vi "Get Output DMA Refs.vi"(8 "error in (no error)":errorcluster, 9 "FPGA Ref":refnum<k20>, 10 "Item GUID":string, 11 "Section Ref in":T7 format="%.0x") -> (0 "error out":errorcluster, 1 "FPGA Ref":refnum<k20>, 2 "DMA":T1[](array[typedef]) {"DMA Settings"."dt" format="%#_p"; "DMA Settings"."Update Rate" items=["1 Hz"=1, "2 Hz"=2, "5 Hz"=5, "10 Hz"=10]; "Refs"."Pairs"."Refs" format="%.0x"}, 3 "Section Ref out":T7 format="%.0x")   [LabVIEW 2013, in "FPGA Addon Engine.lvlib"]
uses:
  FPGA Addon Engine.lvlib
  <vilib>/NI Veristand/Custom Device API/Custom Device Item Ref.ctl
  Types/DMA Output Settings.ctl
  Inline Async API/Controls/Write To VS Engine.ctl
  <vilib>/NI Veristand/Custom Device API/Data Reference.ctl
  Types/DMA Output Ref.ctl
  <vilib>/NI VeriStand/Custom Device Waveform API/Single Waveform Read (DBL)/Single Waveform Read (DBL).lvclass
  Shared/DMA Settings.ctl
  Shared/Delacing Scheme.ctl
  Shared/FG Action.ctl
  <vilib>/NI/LVFPGA Adv Session Resources/OpenByNameSubVI.vi
  <vilib>/rvi/interface/common/niFpgaWaitOnOcc.vi
  <vilib>/NI Veristand/Custom Device Tools/Custom Device Utility Library/NI VeriStand - Search for Item by GUID.vi
  Shared/Constants.vi
  <vilib>/NI Veristand/Custom Device API/Get Item Property (Variant).vi
  <vilib>/NI Veristand/Custom Device Tools/Custom Device Utility Library/NI VeriStand - Search for All Items by GUID.vi
  <vilib>/NI Veristand/Custom Device API/Get Item Property (String).vi
  <vilib>/NI Veristand/Custom Device Waveform API/Single Waveform Read (DBL)/NI VeriStand - Open Single Waveform Read Session (DBL).vi
  <vilib>/NI Veristand/Custom Device API/Get Item Property (Dependent Node Pointer).vi
  <vilib>/rvi/interface/common/dynamic/niFpgaEscapeDelimiterAndNull.vi
  <vilib>/Utility/error.llb/Error Cluster From Error Code.vi
  <vilib>/NI/LVFPGA Adv Session Resources/OpenByName.xnode
  <vilib>/rvi/interface/nirviMethod/nirviMethod.xnode
  Shared/FPGA Addon Shared.lvlib
  <vilib>/NI VeriStand/Custom Device API/Custom Device API.lvlib
  <vilib>/NI Veristand/Custom Device Tools/Custom Device Utility Library/Custom Device Utility Library.lvlib
  <vilib>/NI VeriStand/Custom Device Waveform API/NI_VS Custom Device Waveform API.lvlib
  <vilib>/rvi/errors/niLvFpgaMergeErrorWithErrorCode.vi
  Inline Async API/Inline Async API.lvlib
  <vilib>/FPGAPlugInAG/Dynamic/niLvFpga_StartFifo_Dynamic.vi
  <vilib>/NI/LVFPGA Adv Session Resources/LVFPGAAdvSessionResources.lvlib
  <vilib>/FPGAPlugInAG/Dynamic/niLvFpga_ConfigureFifo_Dynamic.vi
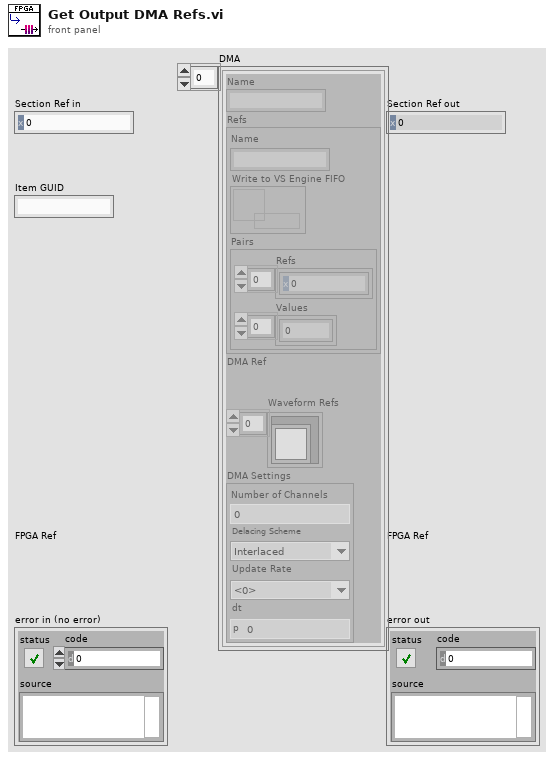
[diagram p1: front panel]
types:
  T1 = typedef "FPGA Addon Engine.lvlib/DMA Output Settings.ctl" = cluster{"Name":string, "Refs":T2, "DMA Ref":T4, "Waveform Refs":refnum<class "Single Waveform Read (DBL).lvclass">[], "DMA Settings":T5}
  T2 = typedef "FPGA Addon Engine.lvlib/Inline Async API.lvlib/Write To VS Engine.ctl" = cluster{"Name":string, "Write to VS Engine FIFO":refnum<k33>, "Pairs":cluster{"Refs":T3[], "Values":dbl[]}}
  T3 = typedef "Custom Device API.lvlib/Data Reference.ctl" = i32
  T4 = typedef "FPGA Addon Engine.lvlib/DMA Output Ref.ctl" = refnum<k20>
  T5 = typedef "FPGA Addon Shared.lvlib/DMA Settings.ctl" = cluster{"Number of Channels":u8, "Delacing Scheme":T6, "Update Rate":u32, "dt":dbl}
  T6 = typedef "FPGA Addon Shared.lvlib/Delacing Scheme.ctl" = enum8{"Interlaced"}
  T7 = typedef "Custom Device API.lvlib/Custom Device Item Ref.ctl" = u64
  T8 = typedef "FPGA Addon Shared.lvlib/FG Action.ctl" = enum8{"GET", "SET"}
  T9 = typedef "Fifo_DMA_Config.ctl" = cluster{"Name":string, "Depth":u32, "Write? (Deprecated:Use Implementation)":bool, "Physical Channel":u32, "Base Address":u32, "Data Width":u32, "Data Type":T10, "FXP Properties":variant, "Write Window Address":u32, "Implementation":T11, "Control Set":u32}
  T10 = typedef "niFpgaDataTypeControl.ctl" = enum32{"Boolean", "I8", "I16", "I32", "I64", "U8", "U16", "U32", "U64", "FXP", "CustomControl", "SGL"}
  T11 = typedef "niFpgaDmaChannelImplementation.ctl" = enum16{"niFpgaTargetToHost", "niFpgaHostToTarget", "niFpgaPeerToPeerWriter", "niFpgaPeerToPeerReader", "niCoreTargetToHost", "niCoreHostToTarget"}
  T12 = cluster{"Name":string, "Depth":u32, "Write? (Deprecated:Use Implementation)":bool, "Physical Channel":u32, "Base Address":u32, "Data Width":u32, "Data Type":enum32{"Boolean", "I8", "I16", "I32", "I64", "U8", "U16", "U32", "U64", "FXP", "CustomControl", "SGL"}, "FXP Properties":variant, "Write Window Address":u32, "Implementation":enum16{"niFpgaTargetToHost", "niFpgaHostToTarget", "niFpgaPeerToPeerWriter", "niFpgaPeerToPeerReader", "niCoreTargetToHost", "niCoreHostToTarget"}, "Control Set":u32}[]
  T13 = cluster{"Name":string, "type":variant, "indicator?":bool}[]
  T14 = typedef "Custom Device API.lvlib/Waveform Data Reference.ctl" = i32
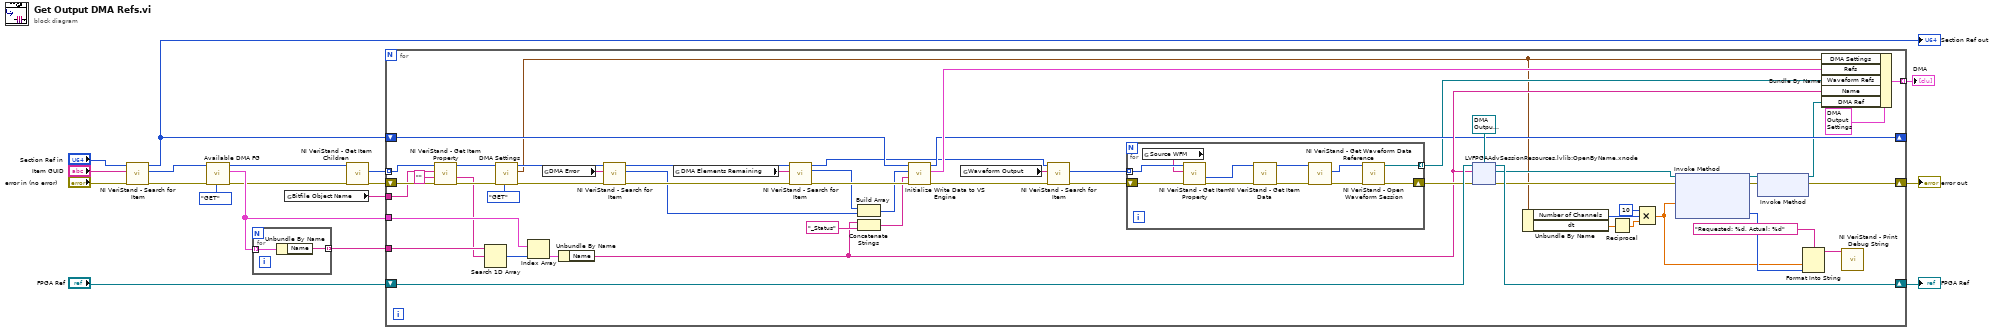
[diagram p0: block diagram]
diagram:
  n1 = call-poly <vilib>:"NI VeriStand - Search for Item.vi"("error in"="error in (no error)", "Item GUID"="Item GUID", "Section Ref in"="Section Ref in") -> ("error out"=w15:errorcluster, "Item Ref"=w17:T7, "Section Ref out"=w2:T7)  [unwired: 5 in, 1 out]
  "Section Ref out" <- w2
  n2 = call "Available DMA FG.vi"("Action"=FG_Action."GET", "error in (no error)"=w15, "Item Ref"=w17) -> ("error out"=w11:errorcluster, "Available DMA"=w12:T9[], "Item Ref out"=w13:T7)  [unwired: 6 in]
  n3 = for {
    tunnel: w12 -> [w20] mode=indexing
    tunnel: [w19] -> w10 mode=indexing
    n4 = Unbundle By Name(w20) -> ("Name"=w19:string)
  }
  n5 = global read "Constants.vi" "Bitfile Object Name"() -> (w9:string)
  n6 = call <vilib>:"NI VeriStand - Get Item Children.vi"("error in (no error)"=w11, "Item Ref in"=w13) -> ("error out"=w7:errorcluster, "Child Refs"=w8:T7[])  [unwired: 6 in, 2 out]
  n7 = for {
    shift-right: [w52] -> w3
    shift-left: w7 -> [w75]
    tunnel: w8 -> [w74] mode=indexing
    tunnel: w9 -> [w73]
    tunnel: w10 -> [w71]
    tunnel: w12 -> [w70]
    shift-right: [w64] -> w4
    shift-left: "FPGA Ref" -> [w65]
    tunnel: [w62] -> w1 mode=indexing
    shift-right: [w30] -> _
    shift-left: w2 -> [w31]
    n8 = call-poly <vilib>:"NI VeriStand - Get Item Property.vi"("error in (no error)"=w75, "Default Value"="", "Property Name"=w73, "Item Ref in"=w74) -> ("error out"=w61:errorcluster, "Value"=w56:string, "Item Ref out"=w60:T7)  [unwired: 4 in, 1 out]
    n9 = Search 1D Array(1D array=w71, element=w56) -> (index of element=w69:i32)  [unwired: 1 in]
    n10 = call "DMA Settings.vi"("Action"=FG_Action."GET", "error in (no error)"=w61, "Item Ref"=w60) -> ("error out"=w45:errorcluster, "DMA Settings"=w27:T5, "Item Ref out"=w44:T7)  [unwired: 6 in]
    n11 = Index Array(array=w70, index=w69) -> (element=w67:T9)
    n12 = global read "Constants.vi" "DMA Error"() -> (w46:string)
    n13 = Unbundle By Name(w67) -> ("Name"=w34:string)
    n14 = call-poly <vilib>:"NI VeriStand - Search for Item.vi"("error in"=w45, "Item GUID"=w46, "Section Ref in"=w44) -> ("error out"=w42:errorcluster, "Item Ref"=w38:T7, "Section Ref out"=w41:T7)  [unwired: 5 in, 1 out]
    n15 = global read "Constants.vi" "DMA Elements Remaining"() -> (w43:string)
    n16 = call-poly <vilib>:"NI VeriStand - Search for Item.vi"("error in"=w42, "Item GUID"=w43, "Section Ref in"=w41) -> ("error out"=w40:errorcluster, "Item Ref"=w37:T7, "Section Ref out"=w29:T7)  [unwired: 5 in, 1 out]
    n17 = Build Array(w37, w38) -> (w36:T7[])
    n18 = Concatenate Strings(w34, "_Status" ("FIFO Name")) -> (w33:string)
    n19 = call "Initialize Write Data to VS Engine.vi"("error in (no error)"=w40, "FIFO Name"=w33, "Hardware Output Refs"=w36, "Device Ref"=w31) -> ("error out"=w39:errorcluster, "Write to VS Engine"=w32:T2, "Device Ref out"=w30:T7)  [unwired: 5 in]
    n20 = global read "Constants.vi" "Waveform Output"() -> (w57:string)
    n21 = call-poly <vilib>:"NI VeriStand - Search for Item.vi"("error in"=w39, "Item GUID"=w57, "Section Ref in"=w29) -> ("error out"=w58:errorcluster, "Item Refs"=w25:T7[])  [unwired: 5 in, 2 out]
    n22 = for {
      shift-right: [w86] -> w59
      shift-left: w58 -> [w82]
      tunnel: [w83] -> w28 mode=indexing
      tunnel: w25 -> [w81] mode=indexing
      n23 = global read "Constants.vi" "Source WFM"() -> (w80:string)
      n24 = call-poly <vilib>:"NI VeriStand - Get Item Property.vi"("error in (no error)"=w82, "Property Name"=w80, "Item Ref in"=w81) -> ("error out"=w79:errorcluster, "Dependent Node Ref"=w77:T7)  [unwired: 5 in, 2 out]
      n25 = call <vilib>:"NI VeriStand - Get Item Data.vi"("error in (no error)"=w79, "Item Ref in"=w77) -> ("error out"=w78:errorcluster, "Item Ref out"=w76:T7)  [unwired: 8 out]
      n26 = call <vilib>:"NI VeriStand - Get Waveform Data Reference.vi"("error in (no error)"=w78, "Waveform Ref in"=w76) -> ("error out"=w85:errorcluster, "Waveform Data Reference"=w84:T14)  [unwired: 7 in, 1 out]
      n27 = call-poly <vilib>:"NI VeriStand - Open Waveform Session.vi"("error in (no error)"=w85, "DBL Waveform Data Reference"=w84) -> ("error out"=w86:errorcluster, "Single Waveform Read Session (DBL)"=w83:refnum<class "Single Waveform Read (DBL).lvclass">)  [unwired: 8 in]
    }
    n28 = xnode "LVFPGAAdvSessionResources.lvlib:OpenByName.xnode"("FPGA VI Reference in"=w65, "Resource name in"=w34, "Single resource reference type in"=T4 refnum, "Error in"=w59) -> ("Single resource reference out"=w51:T4, "Error out"=w53:errorcluster, "FPGA VI Reference out"=w64:refnum<k20>)
    n29 = Unbundle By Name(w27) -> ("Number of Channels"=w48:u8, "dt"=w50:dbl)
    n30 = Reciprocal(x=w50) -> (1/x=w49:dbl)
    n31 = Compound Arithmetic op=MULTIPLY(u8 10 ("value"), w48, w49) -> (w21:dbl)
    n32 = xnode "Invoke Method"("FPGA VI Reference In"=w51, "error in"=w53, "Requested Depth"=w21) -> ("FPGA VI Reference Out"=w55:T4, "error out"=w54:errorcluster, "Actual Depth"=w22:u32)
    n33 = xnode "Invoke Method"("FPGA VI Reference In"=w55, "error in"=w54) -> ("FPGA VI Reference Out"=w26:T4, "error out"=w52:errorcluster)
    n34 = Format Into String(format string="Requested: %d, Actual: %d", w21, w22) -> (resulting string=w24:string)  [unwired: 2 in, 1 out]
    n35 = Bundle By Name(cluster=T1 {"Name"="", "Refs"={"Name"="", "Write to VS Engine FIFO"=refnum, "Pairs"={"Refs"=[], "Values"=[]}}, "DMA Ref"=refnum, "Waveform Refs"=[], "DMA Settings"={"Number of Channels"=0, "Delacing Scheme"=enum."Interlaced", "Update Rate"=0, "dt"=0.0}}, "DMA Settings"=w27, "Refs"=w32, "Waveform Refs"=w28, "Name"=w34, "DMA Ref"=w26) -> (w62:T1)
    n36 = call <vilib>:"NI VeriStand - Print Debug String.vi"("Message"=w24) -> ()  [unwired: 10 in, 1 out]
  }
  "error out" <- w3
  "FPGA Ref" <- w4
  "DMA" <- w1
